vi "dfd_nMAC_CircSubNwEn.vi"(1 "len":fxp<+,16,16>, 2 "idxIn":fxp<+,16,16>, 3 "Enable":bool, 4 "step":fxp<+,16,16>) -> (6 "opWrap?":bool, 7 "idxOut":fxp<+,16,16>)   [LabVIEW 2017]
doc: "opWrap is NOT cleared even if Enable==False."
uses:
  <vilib>/rvi/FXPMathLib/basic elements/FxpAddSub/XNode/nifxpmath_AddSub.xnode
  <vilib>/rvi/FXPMathLib/sim/FxpSim.dll
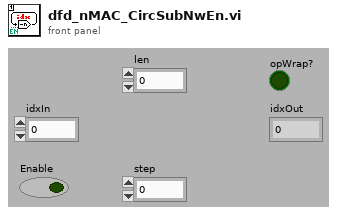
[diagram p1: front panel]
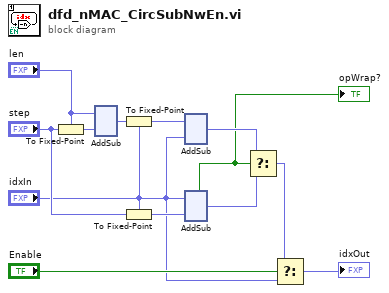
[diagram p0: block diagram]
diagram:
  n1 = To Fixed-Point(fixed-point type="len", number="step") -> (fixed-point=w5:fxp<+,16,16>)
  n2 = xnode "AddSub"("x"="len", "y"=w5) -> ("s"=w6:fxp<+,16,16>)  [unwired: 1 out]
  n3 = To Fixed-Point(fixed-point type="idxIn", number=w6) -> (fixed-point=w3:fxp<+,16,16>)
  n4 = To Fixed-Point(fixed-point type="idxIn", number="step") -> (fixed-point=w2:fxp<+,16,16>)
  n5 = xnode "AddSub"("x"=w3, "y"="idxIn") -> ("s"=w13:fxp<+,16,16>)  [unwired: 1 out]
  n6 = xnode "AddSub"("x"="idxIn", "y"=w2) -> ("s"=w12:fxp<+,16,16>, "borrow-out"=w11:bool)
  "opWrap?" <- w11
  n7 = Select(t=w13, s=w11, f=w12) -> (s? t:f=w9:fxp<+,16,16>)
  n8 = Select(t=w9, s="Enable", f="idxIn") -> (s? t:f=→"idxOut":fxp<+,16,16>)
